vi "matrix multiplication.vi"() -> ()   [LabVIEW 2011]
uses:
  <vilib>/imath/engines/lvmath2/RunTimeEngine/NodeEndStatement/NIMS_NodeEndStatement_Output.vi
  <vilib>/imath/engines/lvmath2/RunTimeEngine/ErrorHandling/NIMS_Finalize Error.vi
panel:
  out "c":i32[][](array[numeric])
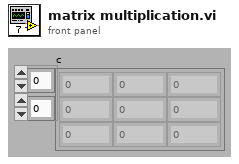
[diagram p1: front panel]
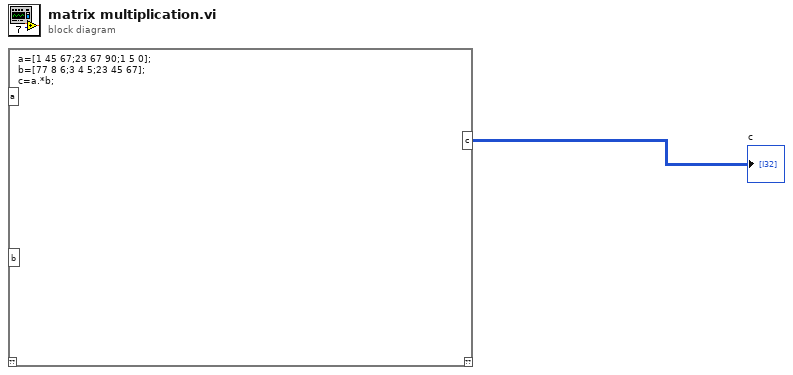
[diagram p0: block diagram]
diagram:
  n1 = mathscript code="a=[1 45 67;23 67 90;1 5 0];\nb=[77 8 6;3 4 5;23 45 67];\nc=a.*b;"() -> ("c"=→"c":i32[][])  [unwired: 3 in, 1 out]
